vi "CRYOne Check.vi"(4 "In":bool[](array[boolean])) -> (1 "Out":bool[](array[boolean]))   [LabVIEW 2013]
panel:
  in  "Single Check?":bool
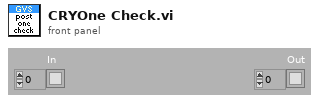
[diagram p1: front panel]
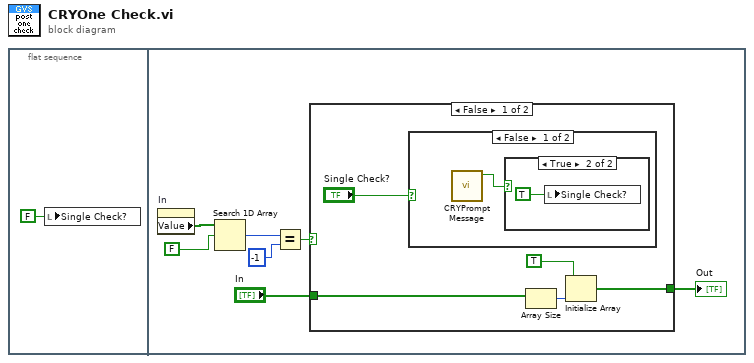
[diagram p0: block diagram]
diagram:
  n1 = flat-sequence {
    frame #0 {
      n2 = local write "Single Check?"(FALSE ("Single Check?")) -> ()
    }
    frame #1 {
      n3 = property on="In" class="Arr (strict)"() -> ("Value"=w8:bool[])  [unwired: 2 in, 2 out]
      n4 = Search 1D Array(1D array=w8, element=FALSE) -> (index of element=w6:i32)  [unwired: 1 out]
      n5 = Equal?(x=w6, y=-1) -> (x = y?=w4:bool)
      n6 = case shown="False" w4 {
        tunnel: [w11 w16] -> w3
        tunnel: "In" -> [w10 w16]
        frame False {
          n7 = case shown="False" "Single Check?" {
            frame False {
              n8 = call "CRYPrompt Message.vi"() -> ("Out"=w14:bool)  [unwired: 2 in, 9 out]
              n9 = case shown="True" w14 {
                frame False {
                }
                frame True {
                  n10 = local write "Single Check?"(TRUE ("Single Check?")) -> ()
                }
              }
            }
            frame True {
            }
          }
          n11 = Array Size(array=w10) -> (size(s)=w13:i32)
          n12 = Initialize Array(TRUE, w13) -> (w11:bool[])
        }
        frame True {
        }
      }
      "Out" <- w3
    }
  }
